vi "Read Gyro.vi"(8 "error in (no error)":errorcluster, 11 "LSM9DS1 IMU in":refnum<class "LSM9DS1 IMU.lvclass">) -> (0 "error out":errorcluster, 2 "Gyro Values (dps)":T1, 3 "LSM9DS1 IMU out":refnum<class "LSM9DS1 IMU.lvclass">)   [LabVIEW 2020, in "LSM9DS1 IMU.lvclass"]
uses:
  LSM9DS1 IMU.lvclass
  3 Axis Values.ctl
  LSM9DS1 IMU.lvclass/LSM9DS1 IMU.ctl
  Read Accel & Gyro I2C.vi
  Write Accel & Gyro I2C.vi
  Read Gyro Range.vi
  LINX I2C/LINX I2C.lvclass
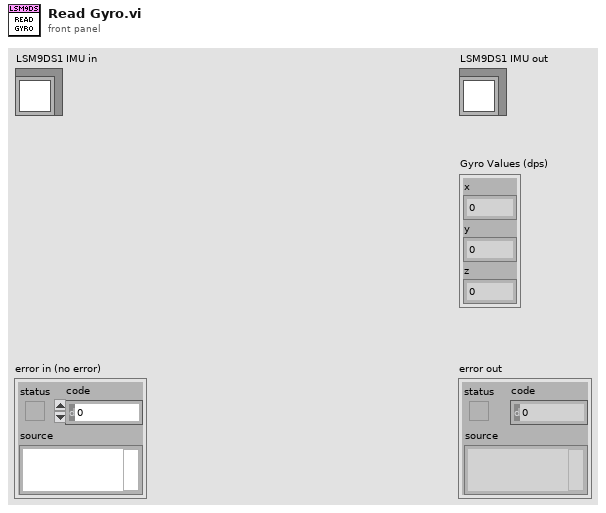
[diagram p1: front panel]
types:
  T1 = typedef "LSM9DS1 IMU.lvclass/3 Axis Values.ctl" = cluster{"x":dbl, "y":dbl, "z":dbl}
  T2 = typedef "LSM9DS1 IMU.lvclass/Gyro Range.ctl" = enum16{"245dps", "500dps", "2000dps"}
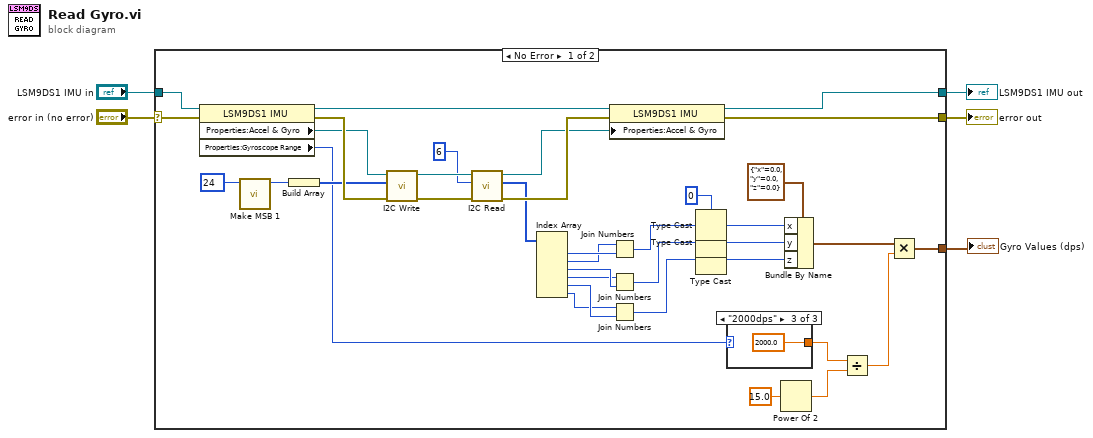
[diagram p0: block diagram]
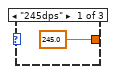
[diagram p2: hidden frame]
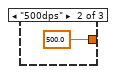
[diagram p3: hidden frame]
diagram:
  n1 = case shown="No Error" "error in (no error)" {
    selector: "error in (no error)" -> [w32 w47]
    tunnel: [w33 w47] -> w4
    tunnel: [w37 w46] -> w2
    tunnel: "LSM9DS1 IMU in" -> [w42 w46]
    tunnel: [w7 _] -> w1
    frame No Error {
      w13 = i16 0
      n2 = property class="LSM9DS1 IMU"(reference=w42, error in=w32) -> (reference out=w38:refnum<class "LSM9DS1 IMU.lvclass">, error out=w36:errorcluster, "Properties:Accel & Gyro"=w31:refnum<class "LINX I2C.lvclass">, "Properties:Gyroscope Range"=w6:T2)
      n3 = call "Make MSB 1.vi"("Register Address"=u8 24) -> ("Register Address | 0x80"=w21:u8)  [unwired: 10 in]
      n4 = Build Array(w21) -> (w20:u8[])
      n5 = call "I2C Write.vi"("error in (no error)"=w36, "Bytes to Write"=w20, "LINX I2C in"=w31) -> ("error out"=w41:errorcluster, "LINX I2C out"=w40:refnum<class "LINX I2C.lvclass">)  [unwired: 7 in]
      n6 = call-dynamic "I2C Read.vi"("error in (no error)"=w41, "# Bytes to Read"=u8 6, "LINX I2C in"=w40) -> ("error out"=w35:errorcluster, "Bytes Read"=w29:u8[], "LINX I2C out"=w30:refnum<class "LINX I2C.lvclass">)  [unwired: 6 in]
      n7 = Index Array(array=w29) -> (element #1=w28:u8, element #2=w27:u8, element #3=w26:u8, element #4=w25:u8, element #5=w24:u8, element #6=w23:u8)  [unwired: 6 in]
      n8 = property class="LSM9DS1 IMU"(reference=w38, error in=w35, "Properties:Accel & Gyro"=w30) -> (reference out=w37:refnum<class "LSM9DS1 IMU.lvclass">, error out=w33:errorcluster)
      n9 = Join Numbers(hi=w27, lo=w28) -> ((hi.lo)=w19:u16)
      n10 = Join Numbers(hi=w25, lo=w26) -> ((hi.lo)=w17:u16)
      n11 = Join Numbers(hi=w23, lo=w24) -> ((hi.lo)=w15:u16)
      n12 = Type Cast(type=w13, x=w19) -> (*(type *) &x=w18:i16)
      n13 = Type Cast(type=w13, x=w17) -> (*(type *) &x=w16:i16)
      n14 = Type Cast(type=w13, x=w15) -> (*(type *) &x=w14:i16)
      n15 = case shown="\"2000dps\"" w6 {
        tunnel: [245.0 500.0 2000.0] -> w10
        frame "245dps" {
        }
        frame "500dps" {
        }
        frame "2000dps" {
        }
      }
      n16 = Power Of 2(x=15.0) -> (2^x=w11:dbl)
      n17 = Bundle By Name(cluster=T1 {"x"=0.0, "y"=0.0, "z"=0.0} ("Gyro Values"), "x"=w18, "y"=w16, "z"=w14) -> (w8:T1)
      n18 = Divide(x=w10, y=w11) -> (x/y=w9:dbl)
      n19 = Multiply(x=w8, y=w9) -> (x*y=w7:T1)
    }
    frame Error {
    }
  }
  "error out" <- w4
  "LSM9DS1 IMU out" <- w2
  "Gyro Values (dps)" <- w1
